vi "getSubArray.vi"(7 "element":string, 11 "all rows 2":string[][](array[string])) -> (3 "Array out":dbl[](array[numeric]))   [LabVIEW 2011]
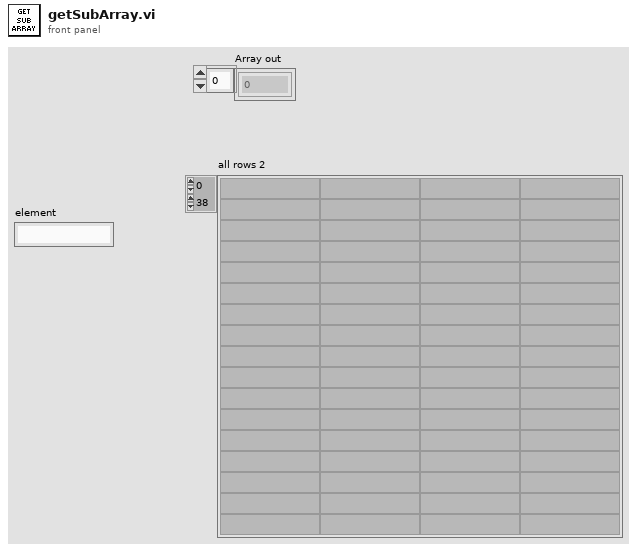
[diagram p1: front panel]
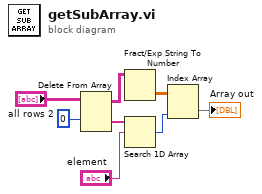
[diagram p0: block diagram]
diagram:
  n1 = Delete From Array(array="all rows 2", index (row)=0) -> (deleted portion=w2:string[], array with subset deleted=w5:string[][])  [unwired: 2 in]
  n2 = Fract/Exp String To Number(string=w5) -> (number=w1:dbl[][])  [unwired: 3 in, 1 out]
  n3 = Search 1D Array(1D array=w2, element="element") -> (index of element=w7:i32)  [unwired: 1 in]
  n4 = Index Array(array=w1, index (col)=w7) -> (element=→"Array out":dbl[])  [unwired: 1 in]
